vi "Check Tw less than Tw_max.vi"(2 "T0 (°C)":dbl=20.0, 3 "Tw max (°C)":dbl=300.0, 4 "alpha0 (/°C)":dbl=0.0036, 5 "Overheat ratio (Rw / R0)":dbl=1.7) -> (0 "Tw < Tw_max":bool=TRUE, 1 "Tw (°C)":dbl=214.44444444444443)   [LabVIEW 2020]
doc: "Calculate wire temperature Tw and check that it is less than the maximum allowable.\nPN 06-NOV-23."
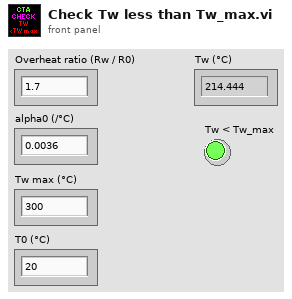
[diagram p1: front panel]
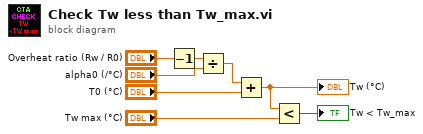
[diagram p0: block diagram]
diagram:
  n1 = Decrement(x="Overheat ratio (Rw / R0)") -> (x-1=w6:dbl)
  n2 = Divide(x=w6, y="alpha0 (/°C)") -> (x/y=w4:dbl)
  n3 = Add(x=w4, y="T0 (°C)") -> (x+y=w2:dbl)
  "Tw (°C)" <- w2
  n4 = Less?(x=w2, y="Tw max (°C)") -> (x < y?=→"Tw < Tw_max":bool)
